vi "Read DC Motor Velocities.vi"(8 "error in (no error)":errorcluster, 11 "starter kit host in":refnum<class "NI_Robotics_Starter Kit Host.lvclass">) -> (0 "error out":errorcluster, 1 "right motor ccw velocity (rad/s)":dbl, 2 "left motor ccw velocity (rad/s)":dbl, 3 "starter kit host out":refnum<class "NI_Robotics_Starter Kit Host.lvclass">)   [LabVIEW 2017, in "NI_Robotics_Starter Kit Host.lvclass"]
doc: "<B>Owning Palette:</B> Starter Kit 1.0 VIs, Starter Kit 2.0 VIs\n\nReads and returns the velocities of the left and right drive motors on the Starter Kit robot in the counterclockwise direction. The left and right motors are defined by their positions as you view the robot from behind."
uses:
  <vilib>/robotics/Starter Kit/Host Interface/NI_Robotics_Starter Kit Host.lvclass
  <vilib>/robotics/Starter Kit/Host Interface/NI_Robotics_Starter Kit Host.lvclass/NI_Robotics_Starter Kit Host.ctl
  <instrlib>/DC Motor Controller/HAIOL/DC Motor Controller.lvclass
  <vilib>/robotics/Utilities/NI_Robotics Utilities.lvlib
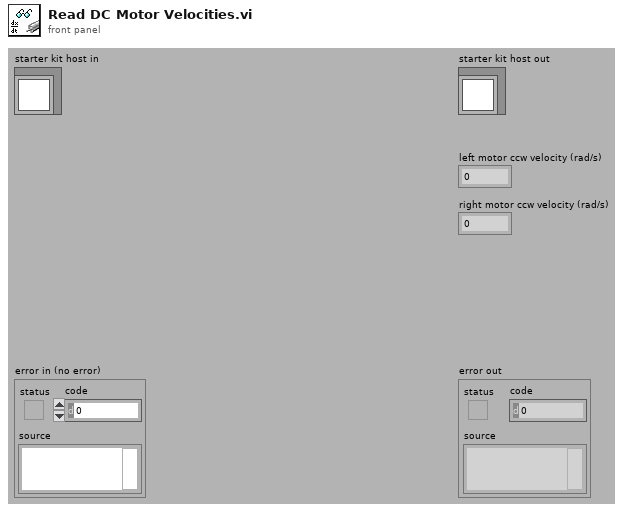
[diagram p1: front panel]
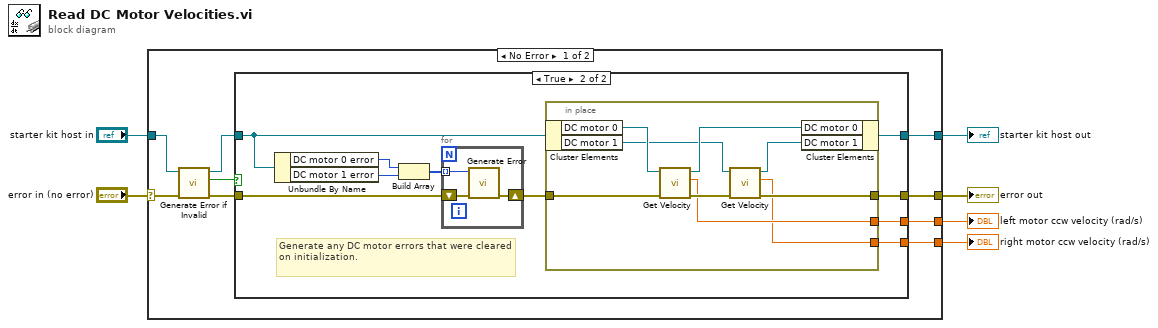
[diagram p0: block diagram]
diagram:
  n1 = case shown="No Error" "error in (no error)" {
    selector: "error in (no error)" -> [w11 w41]
    tunnel: [w15 w41] -> w4
    tunnel: [w14 w40] -> w3
    tunnel: "starter kit host in" -> [w9 w40]
    tunnel: [w13 _] -> w2
    tunnel: [w12 _] -> w1
    frame No Error {
      n2 = call <vilib>:"Generate Error if Invalid.vi"("error in (no error)"=w11, "starter kit host in"=w9) -> ("error out"=w10:errorcluster, "valid?"=w7:bool, "starter kit host out"=w8:refnum<class "NI_Robotics_Starter Kit Host.lvclass">)  [unwired: 7 in]
      n3 = case shown="True" w7 {
        tunnel: [w17 w27] -> w15
        tunnel: [w16 w26] -> w14
        tunnel: [_ w25] -> w13
        tunnel: [_ w24] -> w12
        tunnel: w10 -> [w17 w20]
        tunnel: w8 -> [w16 w23]
        frame False {
        }
        frame True {
          # "Generate any DC motor errors that were cleared on initialization."
          n4 = Unbundle By Name(w23) -> ("DC motor 0 error"=w22:i32, "DC motor 1 error"=w21:i32)
          n5 = Build Array(w22, w21) -> (w18:i32[])
          n6 = for {
            shift-right: [w29] -> w19
            shift-left: w20 -> [w30]
            tunnel: w18 -> [w28] mode=indexing
            n7 = call <vilib>:"Generate Error.vi"("error in (no error)"=w30, "code"=w28) -> ("error out"=w29:errorcluster)  [unwired: 9 in]
          }
          n8 = in-place {
            in-place-border: w19 -> [w39]
            in-place-border: [w33] -> w27
            in-place-border: [w32] -> w25
            in-place-border: [w31] -> w24
            n9 = in-place-cluster #1(w23) -> ("DC motor 0"=w37:refnum<class "DC Motor Controller.lvclass">, "DC motor 1"=w35:refnum<class "DC Motor Controller.lvclass">)
            n10 = call-dynamic "Get Velocity.vi"("error in (no error)"=w39, "DC Motor Controller in"=w37) -> ("error out"=w38:errorcluster, "CCW Velocity (rad/s)"=w32:dbl, "DC Motor Controller out"=w36:refnum<class "DC Motor Controller.lvclass">)  [unwired: 7 in]
            n11 = call-dynamic "Get Velocity.vi"("error in (no error)"=w38, "DC Motor Controller in"=w35) -> ("error out"=w33:errorcluster, "CCW Velocity (rad/s)"=w31:dbl, "DC Motor Controller out"=w34:refnum<class "DC Motor Controller.lvclass">)  [unwired: 7 in]
            n12 = in-place-cluster #1("DC motor 0"=w36, "DC motor 1"=w34) -> (w26:refnum<class "NI_Robotics_Starter Kit Host.lvclass">)
          }
        }
      }
    }
    frame Error {
    }
  }
  "error out" <- w4
  "starter kit host out" <- w3
  "right motor ccw velocity (rad/s)" <- w1
  "left motor ccw velocity (rad/s)" <- w2
